vi "Y-.vi"(8 "Width":dbl=20.0, 9 "Length":dbl=20.0, 10 "Z":dbl, 11 "Y":dbl) -> (0 "Y-":dbl, 3 "(Y-)^2":dbl)   [LabVIEW 2020]
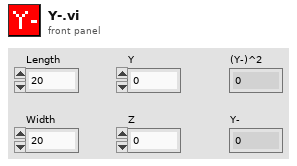
[diagram p1: front panel]
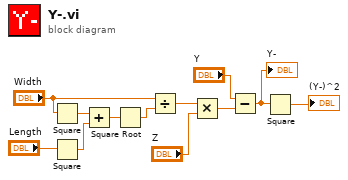
[diagram p0: block diagram]
diagram:
  n1 = Square(x="Width") -> (x^2=w4:dbl)
  n2 = Square(x="Length") -> (x^2=w3:dbl)
  n3 = Add(x=w4, y=w3) -> (x+y=w2:dbl)
  n4 = Square Root(x=w2) -> (sqrt(x)=w5:dbl)
  n5 = Divide(x="Width", y=w5) -> (x/y=w8:dbl)
  n6 = Multiply(x=w8, y="Z") -> (x*y=w10:dbl)
  n7 = Subtract(x="Y", y=w10) -> (x-y=w12:dbl)
  "Y-" <- w12
  n8 = Square(x=w12) -> (x^2=→"(Y-)^2":dbl)
